vi "Test_Manual_BP4610-2.vi"() -> ()   [LabVIEW 2019]
uses:
  _ctrl/create-rw-close.ctl
  _ctrl/BP4610_cmd.ctl
  _ctrl/rw.ctl
  _ctrl/BP4610_return.ctl
  _ctrl/BP4610_config.ctl
panel:
  out "error out":errorcluster
  in  "check":bool
  out "n":i32
  out "BP4610 Err":bool
  in  "BP4610 Config":T1={"VISA"="", "Limit-BP"={"Set"=enum."Current", "Voltage+[V]"=20.0, "Current+[A]"=5.0, "Voltage-[V]"=-20.0, "Current-[A]"=-5.0}, "SET BP"={"Set"=enum."FREQ/WAVE", "Operation mode"=0, "Voltage[Vp-p]"=0.0, "Current[Ap-p]"=0.0, "Voltage[V]"=0.0, "Current[A]"=0.0, "Frequency[Hz]"=1.0, "Waveform"=enum."Sine"}} {"SET BP"."Frequency[Hz]" min=1.0 max=100000.0 step=0.1; "SET BP"."Current[A]" min=-20.0 max=20.0 step=0.001; "SET BP"."Voltage[V]" min=-115.0 max=115.0 step=0.01; "SET BP"."Current[Ap-p]" min=0.0 max=60.0 step=0.01; "SET BP"."Voltage[Vp-p]" min=0.0 max=120.0 step=0.1; "SET BP"."Operation mode" items=["CV-INT", "CV-EXT", "CV-ADD", "CC-INT", "CC-EXT", "CC-ADD"]; "Limit-BP"."Current-[A]" min=-20.0 max=20.0 step=0.001; "Limit-BP"."Voltage-[V]" min=-115.0 max=115.0 step=0.01; "Limit-BP"."Current+[A]" min=0.0 max=60.0 step=0.01; "Limit-BP"."Voltage+[V]" min=0.0 max=120.0 step=0.1}
  out "output":T2 {"DC current[A]" format="%.2f"; "DC voltage[V]" format="%.1f"}
  in  "read":bool
  in  "output":bool
  in  "Exit":bool
  in  "close":bool
  in  "open":bool
  # "NF BP4610"
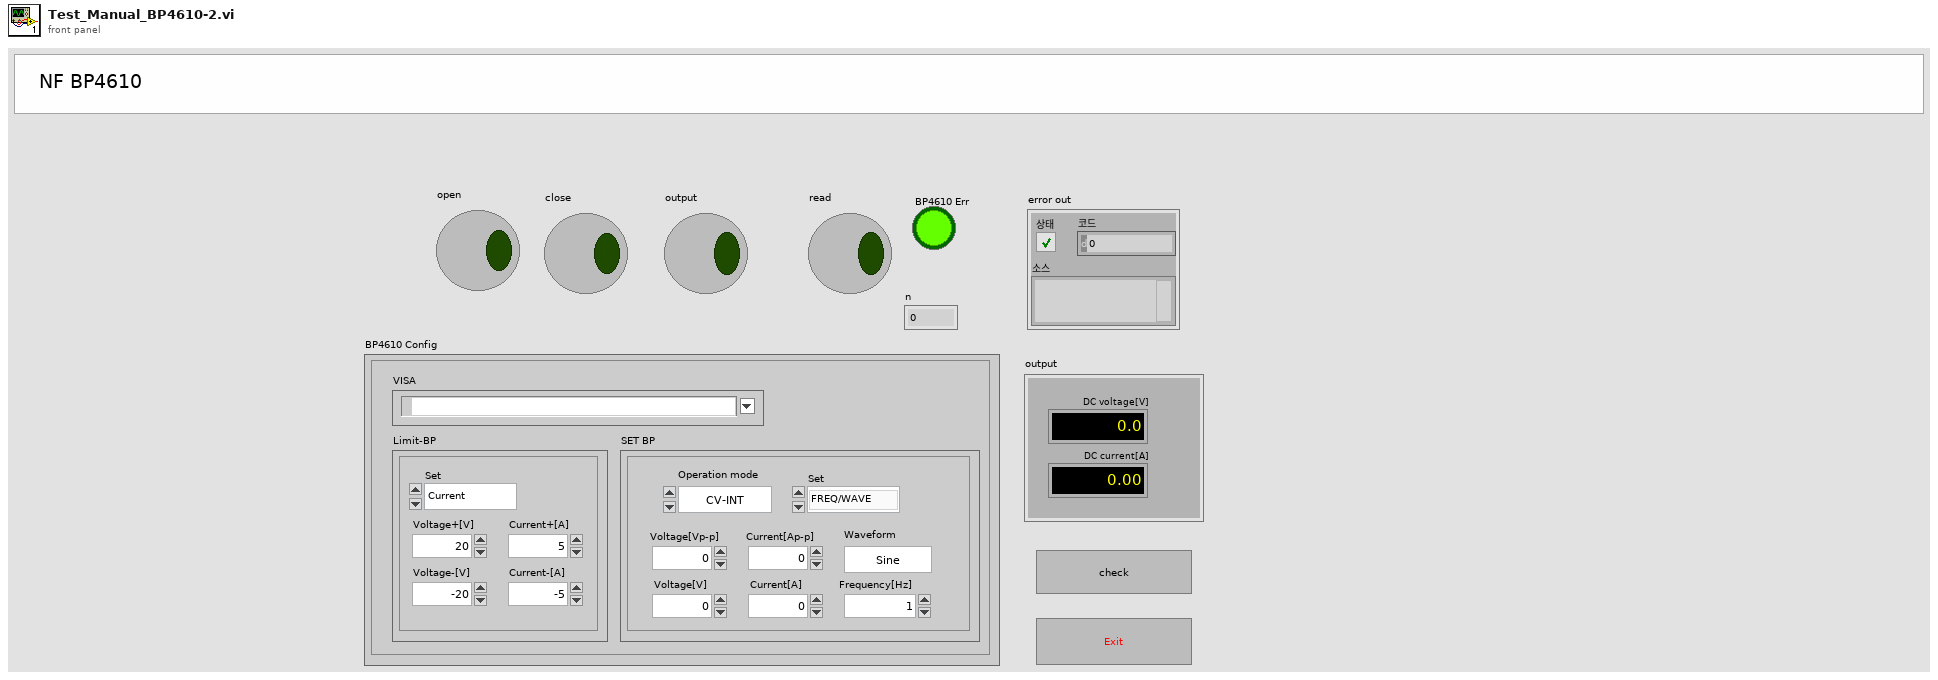
[diagram p1: front panel]
types:
  T1 = typedef "BP4610_config.ctl" = cluster{"VISA":refnum<visa-resource-name>, "Limit-BP":cluster{"Set":enum16{"Current", "Voltage"}, "Voltage+[V]":dbl, "Current+[A]":dbl, "Voltage-[V]":dbl, "Current-[A]":dbl}, "SET BP":cluster{"Set":enum16{"Current", "Voltage", "FREQ/WAVE"}, "Operation mode":u16, "Voltage[Vp-p]":dbl, "Current[Ap-p]":dbl, "Voltage[V]":dbl, "Current[A]":dbl, "Frequency[Hz]":dbl, "Waveform":enum16{"Sine", "Square", "ARB 1", "ARB 2", "ARB 3", "ARB 4", "ARB 5", "ARB 6", "ARB 7", "ARB 8", "ARB 9", "ARB 10", "ARB 11", "ARB 12", "ARB 13", "ARB 14", "ARB 15", "ARB 16"}}}
  T2 = typedef "BP4610_return.ctl" = cluster{"DC voltage[V]":dbl, "DC current[A]":dbl}
  T3 = typedef "rw.ctl" = enum16{"read", "write"}
  T4 = typedef "create-rw-close.ctl" = enum16{"create", "write", "read", "close"}
  T5 = enum8{"Enabled", "Disabled", "Disabled and Grayed Out"}
  T6 = typedef "BP4610_cmd.ctl" = enum16{"open", "read", "set", "limit", "output on", "output off", "close"}
  T7 = typedef "BP4610_cmd.ctl" = enum16{"open", "read", "set", "limit", "output", "close"}
  T8 = typedef "Error list.ctl" = cluster{"DL950":bool, "BP4610":bool, "DSP":bool, "AI":bool, "AO":bool, "DO":bool}
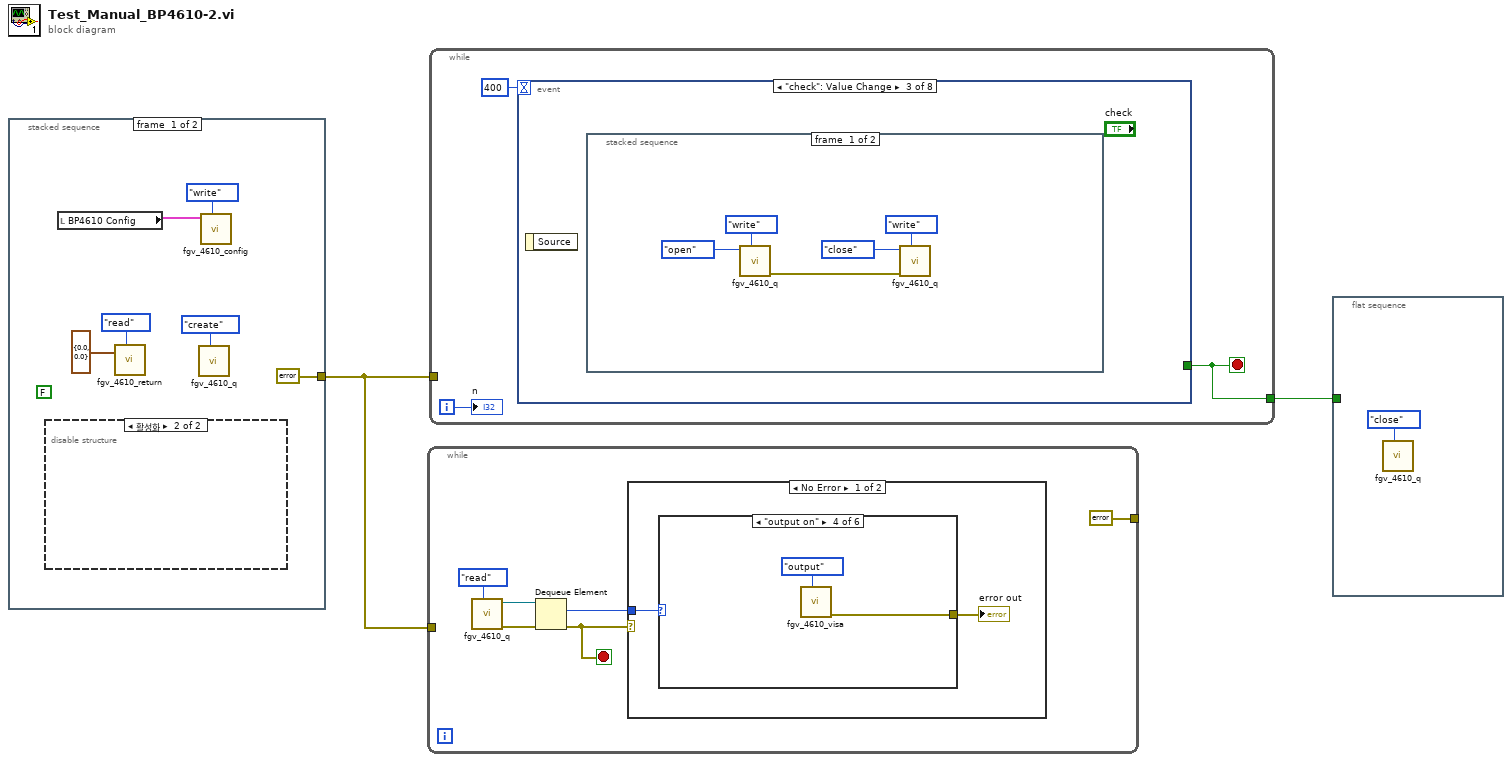
[diagram p0: block diagram]
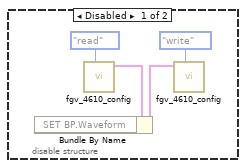
[diagram p2: hidden frame]
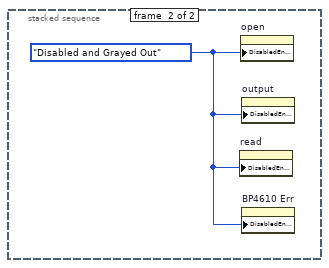
[diagram p3: hidden frame]
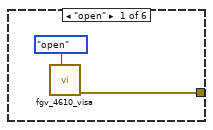
[diagram p4: hidden frame]
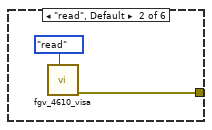
[diagram p5: hidden frame]
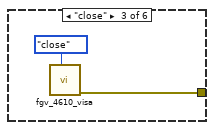
[diagram p6: hidden frame]
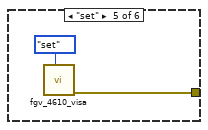
[diagram p7: hidden frame]
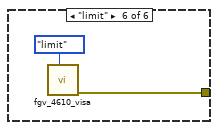
[diagram p8: hidden frame]
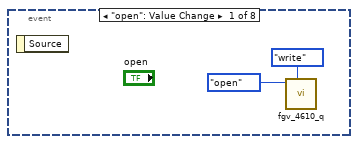
[diagram p10: hidden frame]
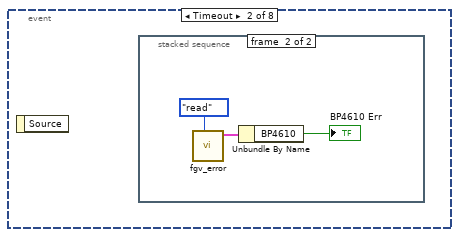
[diagram p11: hidden frame]
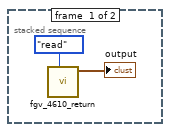
[diagram p12: hidden frame]
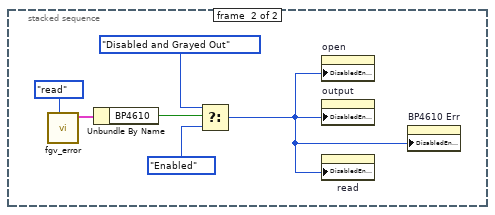
[diagram p13: hidden frame]
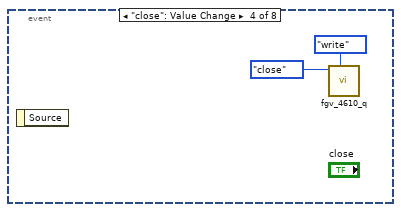
[diagram p14: hidden frame]
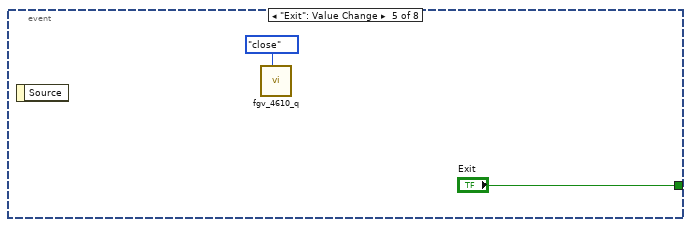
[diagram p15: hidden frame]
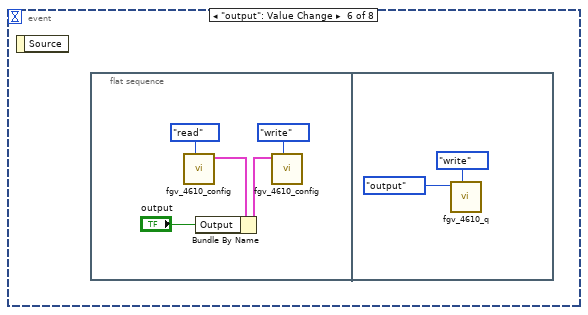
[diagram p16: hidden frame]
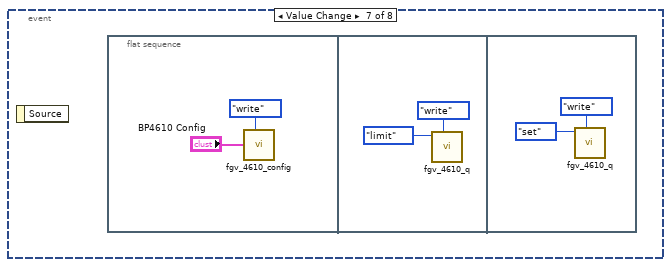
[diagram p17: hidden frame]
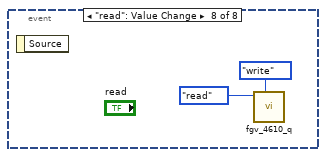
[diagram p18: hidden frame]
diagram:
  n1 = stacked-sequence {
    tunnel: [errorcluster {"status"=FALSE, "code"=0, "source"=""} ("에러 상수") _] -> w2
    frame #0 {
      (unwired) FALSE ("output")
      n2 = disable-structure shown="활성화" {
        frame Disabled {
          n3 = call "fgv_4610_config.vi"("cmd"=rw."read") -> ("BP4610 Config 2"=w10:T1)  [unwired: 9 in, 1 out]
          n4 = Bundle By Name(cluster=w10) -> (w11:T1)  [unwired: 1 in]
          n5 = call "fgv_4610_config.vi"("cmd"=rw."write", "BP4610 Config"=w11) -> ()  [unwired: 8 in, 2 out]
        }
        frame Enabled {
        }
      }
      n6 = local read "BP4610 Config"() -> (w3:T1)
      n7 = call "fgv_4610_return.vi"("cmd"=rw."read", "output"=T2 {"DC voltage[V]"=0.0, "DC current[A]"=0.0}) -> ()  [unwired: 9 in, 1 out]
      n8 = call "fgv_4610_q.vi"("cmd"=create-rw-close."create") -> ()  [unwired: 9 in, 2 out]
      n9 = call "fgv_4610_config.vi"("cmd"=rw."write", "BP4610 Config"=w3) -> ()  [unwired: 8 in, 2 out]
    }
    frame #1 {
      w13 = T5."Disabled and Grayed Out" ("비활성화")
      n10 = property on="read" class="Bool"("DisabledEnum"=w13) -> ()  [unwired: 2 in, 2 out]
      n11 = property on="open" class="Bool"("DisabledEnum"=w13) -> ()  [unwired: 2 in, 2 out]
      n12 = property on="output" class="Bool (strict)"("DisabledEnum"=w13) -> ()  [unwired: 2 in, 2 out]
      n13 = property on="BP4610 Err" class="Bool (strict)"("DisabledEnum"=w13) -> ()  [unwired: 2 in, 2 out]
    }
  }
  n14 = while {
    tunnel: w2 -> [_]
    tunnel: [errorcluster {"status"=FALSE, "code"=0, "source"=""} ("error out")] -> _
    stop <- w15 stop-if-true
    n15 = call "fgv_4610_q.vi"("cmd"=create-rw-close."read") -> ("error out"=w18:errorcluster, "queue out"=w17:refnum<queue>)  [unwired: 9 in]
    n16 = Dequeue Element(queue=w17, error in (no error)=w18) -> (element=w16:T6, error out=w15:errorcluster)  [unwired: 1 in, 2 out]
    n17 = case shown="No Error" w15 {
      tunnel: w16 -> [w21 _]
      frame No Error {
        n18 = case shown="\"output on\"" w21 {
          tunnel: [w22 w24 w26 w28 w30 w32] -> w20
          frame "open" {
            n19 = call "fgv_4610_visa.vi"("cmd"=BP4610_cmd."open") -> ("error out"=w22:errorcluster)  [unwired: 10 in]
          }
          frame "read", Default {
            n20 = call "fgv_4610_visa.vi"("cmd"=BP4610_cmd."read") -> ("error out"=w24:errorcluster)  [unwired: 10 in]
          }
          frame "close" {
            n21 = call "fgv_4610_visa.vi"("cmd"=BP4610_cmd."close") -> ("error out"=w26:errorcluster)  [unwired: 10 in]
          }
          frame "output on" {
            n22 = call "fgv_4610_visa.vi"("cmd"=BP4610_cmd."output") -> ("error out"=w28:errorcluster)  [unwired: 10 in]
          }
          frame "set" {
            n23 = call "fgv_4610_visa.vi"("cmd"=BP4610_cmd."set") -> ("error out"=w30:errorcluster)  [unwired: 10 in]
          }
          frame "limit" {
            n24 = call "fgv_4610_visa.vi"("cmd"=BP4610_cmd."limit") -> ("error out"=w32:errorcluster)  [unwired: 10 in]
          }
        }
        "error out" <- w20
      }
      frame Error {
      }
    }
  }
  n25 = while {
    tunnel: w2 -> [_]
    tunnel: [w36] -> w1
    i -> [w34]
    stop <- w36 stop-if-true
    n26 = event shown="[2] \"check\": Value Change" {
      selector: _ -> [_ _ _ _ _ _ _ _]
      dyn-events: _ -> [_ _ _ _ _ _ _ _]
      timeout: 400 -> [_ _ _ _ _ _ _ _]
      tunnel: [_ _ _ _ "Exit" _ _ _] -> w36
      event "open": Value Change {
        n27 = event-data() -> ()  [unwired: 1 in, 1 out]
        n28 = call "fgv_4610_q.vi"("cmd"=create-rw-close."write", "action"=BP4610_cmd."open") -> ()  [unwired: 8 in, 2 out]
      }
      event Timeout {
        n29 = event-data() -> ()  [unwired: 1 in, 1 out]
        n30 = stacked-sequence {
          frame #0 {
            n31 = call "fgv_4610_return.vi"("cmd"=rw."read") -> ("output 2"=→"output":T2)  [unwired: 10 in]
          }
          frame #1 {
            n32 = call "fgv_error.vi"("cmd"=rw."read") -> ("error cluster 2"=w42:T8)  [unwired: 10 in]
            n33 = Unbundle By Name(w42) -> ("BP4610"=→"BP4610 Err":bool)
          }
        }
      }
      event "check": Value Change {
        n34 = event-data() -> ()  [unwired: 1 in, 1 out]
        n35 = stacked-sequence {
          frame #0 {
            n36 = call "fgv_4610_q.vi"("cmd"=create-rw-close."write", "action"=BP4610_cmd."open") -> ("error out"=w44:errorcluster)  [unwired: 8 in, 1 out]
            n37 = call "fgv_4610_q.vi"("cmd"=create-rw-close."write", "error in"=w44, "action"=BP4610_cmd."close") -> ()  [unwired: 7 in, 2 out]
          }
          frame #1 {
            n38 = call "fgv_error.vi"("cmd"=rw."read") -> ("error cluster 2"=w53:T8)  [unwired: 10 in]
            n39 = Unbundle By Name(w53) -> ("BP4610"=w52:bool)
            n40 = Select(t=T5."Disabled and Grayed Out" ("비활성화"), s=w52, f=T5."Enabled" ("비활성화")) -> (s? t:f=w49:T5)
            n41 = property on="open" class="Bool"("DisabledEnum"=w49) -> ()  [unwired: 2 in, 2 out]
            n42 = property on="output" class="Bool (strict)"("DisabledEnum"=w49) -> ()  [unwired: 2 in, 2 out]
            n43 = property on="read" class="Bool"("DisabledEnum"=w49) -> ()  [unwired: 2 in, 2 out]
            n44 = property on="BP4610 Err" class="Bool (strict)"("DisabledEnum"=w49) -> ()  [unwired: 2 in, 2 out]
          }
        }
      }
      event "close": Value Change {
        n45 = event-data() -> ()  [unwired: 1 in, 1 out]
        n46 = call "fgv_4610_q.vi"("cmd"=create-rw-close."write", "action"=BP4610_cmd."close") -> ()  [unwired: 8 in, 2 out]
      }
      event "Exit": Value Change {
        n47 = event-data() -> ()  [unwired: 1 in, 1 out]
        n48 = call "fgv_4610_q.vi"("cmd"=create-rw-close."close") -> ()  [unwired: 9 in, 2 out]
      }
      event "output": Value Change {
        n49 = event-data() -> ()  [unwired: 1 in, 1 out]
        n50 = flat-sequence {
          frame #0 {
            n51 = call "fgv_4610_config.vi"("cmd"=rw."read") -> ("BP4610 Config 2"=w62:T1)  [unwired: 9 in, 1 out]
            n52 = Bundle By Name(cluster=w62, "Output"="output") -> (w61:T1)
            n53 = call "fgv_4610_config.vi"("cmd"=rw."write", "BP4610 Config"=w61) -> ()  [unwired: 8 in, 2 out]
          }
          frame #1 {
            n54 = call "fgv_4610_q.vi"("cmd"=create-rw-close."write", "action"=BP4610_cmd."output") -> ()  [unwired: 8 in, 2 out]
          }
        }
      }
      event Value Change {
        n55 = event-data() -> ()  [unwired: 1 in, 1 out]
        n56 = flat-sequence {
          frame #0 {
            n57 = call "fgv_4610_config.vi"("cmd"=rw."write", "BP4610 Config"="BP4610 Config") -> ()  [unwired: 8 in, 2 out]
          }
          frame #1 {
            n58 = call "fgv_4610_q.vi"("cmd"=create-rw-close."write", "action"=BP4610_cmd."limit") -> ()  [unwired: 8 in, 2 out]
          }
          frame #2 {
            n59 = call "fgv_4610_q.vi"("cmd"=create-rw-close."write", "action"=BP4610_cmd."set") -> ()  [unwired: 8 in, 2 out]
          }
        }
      }
      event "read": Value Change {
        n60 = event-data() -> ()  [unwired: 1 in, 1 out]
        n61 = call "fgv_4610_q.vi"("cmd"=create-rw-close."write", "action"=BP4610_cmd."read") -> ()  [unwired: 8 in, 2 out]
      }
    }
    "n" <- w34
  }
  n62 = flat-sequence {
    tunnel: w1 -> [_]
    frame #0 {
      n63 = call "fgv_4610_q.vi"("cmd"=create-rw-close."close") -> ()  [unwired: 9 in, 2 out]
    }
  }
